vi "SL_0.vi"   [LabVIEW 2015, in "Lego_Swerve_2015.lvrbt"]
uses:
  Lego_Swerve_2015.lvrbt
  <vilib>/NXT/Block Support/NXT_OutputPort.ctl
  <vilib>/NXT/Block Support/NXT_MessageMailbox.ctl
  <vilib>/NXT/NXTIO Xnodes/NXTIONodeSubVIs/LEGOResetMotors.vi
  <vilib>/NXT/Dual Mode Library/Motors/Rotation.vi
  <vilib>/NXT/NXTIO Xnodes/NXTIONodeSubVIs/LEGOMotorStatus.vi
  <vilib>/NXT/Dual Mode Library/Display/drawNumber.vi
  <vilib>/NXT/Dual Mode Library/BT/BlueTooth_Read_string.vi
  <vilib>/NXT/NXTIO Xnodes/NXTIONodeSubVIs/NXTMoveMotors.vi
  <vilib>/NXT/Dual Mode Library/Display/drawText.vi
  <vilib>/NXT/Subs/LVHSConnector.ctl
  <vilib>/NXT/NXTIO Xnodes/AddressXNode/NXTIOAddress.xnode
  <vilib>/NXT/NXTIO Xnodes/NXTIOXNode/NXTIO.xnode
  <vilib>/NXT/LegoClasses/BrickReference/BrickReference.lvclass
types:
  T1 = typedef "NXT_OutputPort.ctl" = u8
  T2 = typedef "LVHSConnector.ctl" = refnum<class "BrickReference.lvclass">
  T3 = typedef "NXT_MessageMailbox.ctl" = u8
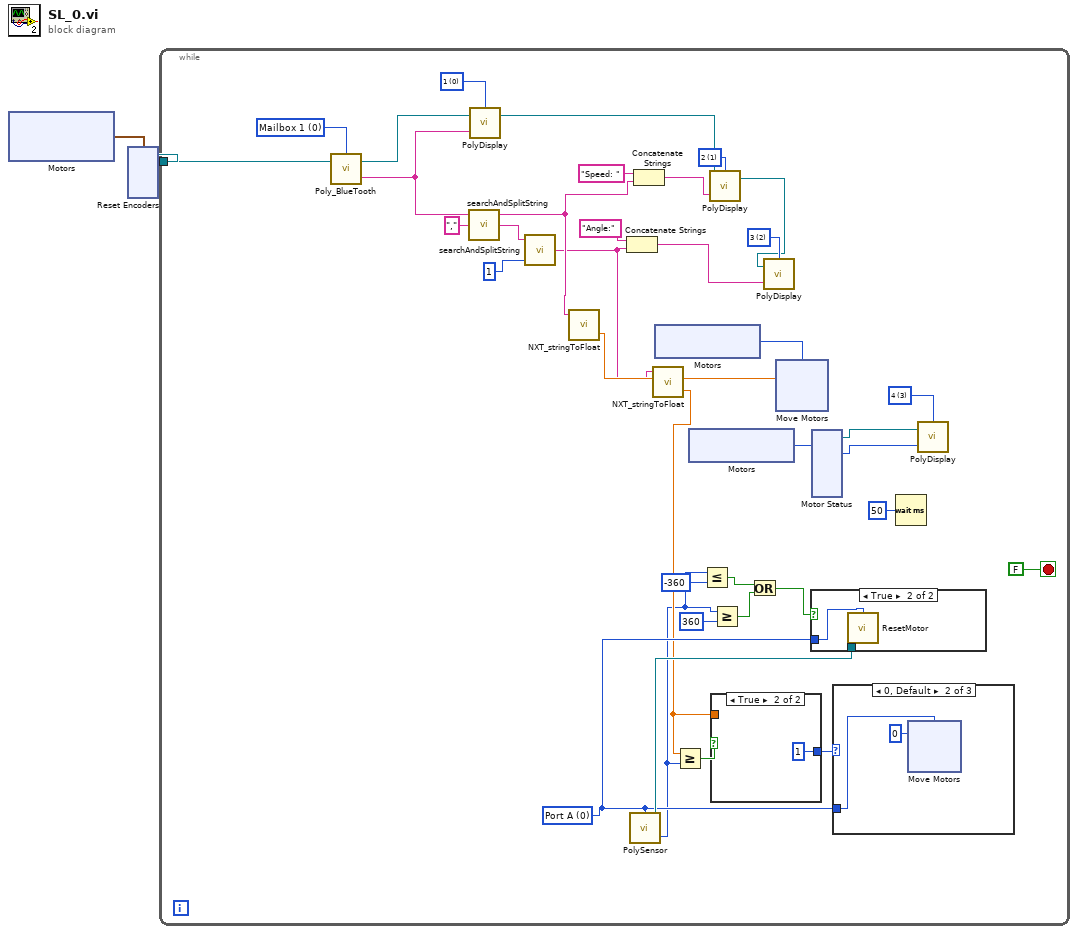
[diagram p0: block diagram]
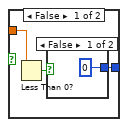
[diagram p2: hidden frame]
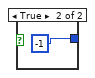
[diagram p3: hidden frame]
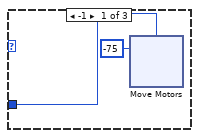
[diagram p5: hidden frame]
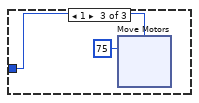
[diagram p6: hidden frame]
diagram:
  n1 = xnode "Motors"() -> ("Motor"=w1:cluster{"Port":T1, "Port":T1})
  n2 = xnode "Reset Encoders"("Motors"=w1) -> ("NXT/EV3"=w2:T2)  [unwired: 1 in]
  n3 = while {
    tunnel: w2 -> [w18]
    stop <- FALSE stop-if-true
    w11 = T1 0 items=["Port A", "Port B", "Port C", "Port D"] ("Port (Port A)")
    w16 = i16 3 items=["1", "2", "3", "4", "5", "6", "7", "8", "9", "10", "11", "12"] ("Line")
    w33 = i16 1 items=["1", "2", "3", "4", "5", "6", "7", "8", "9", "10", "11", "12"] ("Line")
    w34 = i16 2 items=["1", "2", "3", "4", "5", "6", "7", "8", "9", "10", "11", "12"] ("Line")
    w35 = i16 0 items=["1", "2", "3", "4", "5", "6", "7", "8", "9", "10", "11", "12"] ("Line")
    w37 = T3 0 items=["Mailbox 1", "Mailbox 2", "Mailbox 3", "Mailbox 4", "Mailbox 5", "Mailbox 6", "Mailbox 7", "Mailbox 8", "Mailbox 9", "Mailbox 10"] ("Mailbox")
    n4 = call-poly <vilib>:"Poly_BlueTooth.vi"("NXT/EV3"=w18, "Mailbox"=w37) -> ("Message"=w38:string, "NXT/EV3"=w22:T2)  [unwired: 1 in]
    n5 = call <vilib>:"searchAndSplitString.vi"("search string/char (-)"=",", "string"=w38) -> ("match + rest of string"=w26:string, "substring before match"=w25:string)  [unwired: 1 in, 1 out]
    n6 = call-poly <vilib>:"PolyDisplay.vi"("Text"=w38, "NXT/EV3"=w22, "Line"=w35) -> ("NXT/EV3"=w21:T2)  [unwired: 1 in]
    n7 = call <vilib>:"searchAndSplitString.vi"("offset (0)"=1, "string"=w26) -> ("match + rest of string"=w23:string)  [unwired: 1 in, 2 out]
    n8 = call <vilib>:"NXT_stringToFloat.vi"("string"=w25) -> ("number"=w24:sgl)  [unwired: 2 in, 1 out]
    n9 = Concatenate Strings("Angle:" ("string"), w23) -> (w30:string)
    n10 = call-poly <vilib>:"PolySensor.vi"("Port (Port A)"=w11) -> ("Angle of Rotation"=w4:i32, "NXT/EV3"=w13:T2)  [unwired: 2 in]
    n11 = Concatenate Strings("Speed: " ("string"), w25) -> (w32:string)
    n12 = call <vilib>:"NXT_stringToFloat.vi"("string"=w23) -> ("number"=w8:sgl)  [unwired: 2 in, 1 out]
    n13 = xnode "Motors"() -> ("Motor"=w28:T1)
    n14 = Greater Or Equal?(x=w8, y=w4) -> (x >= y?=w10:bool)
    n15 = xnode "Motors"() -> ("Motor"=w14:T1)
    n16 = Less Or Equal?(x=w4, y=-360) -> (x <= y?=w5:bool)
    n17 = call-poly <vilib>:"PolyDisplay.vi"("Text"=w32, "NXT/EV3"=w21, "Line"=w33) -> ("NXT/EV3"=w20:T2)  [unwired: 1 in]
    n18 = case shown="True" w10 {
      tunnel: [w42 1] -> w9
      tunnel: w8 -> [w40 _]
      frame False {
        n19 = Less Than 0?(x=w40) -> (x < 0?=w41:bool)
        n20 = case shown="False" w41 {
          tunnel: [0 -1] -> w42
          frame False {
          }
          frame True {
          }
        }
      }
      frame True {
      }
    }
    n21 = Greater Or Equal?(x=w4, y=360) -> (x >= y?=w7:bool)
    n22 = Or(x=w5, y=w7) -> (x .or. y?=w6:bool)
    n23 = call-poly <vilib>:"PolyDisplay.vi"("Text"=w30, "NXT/EV3"=w20, "Line"=w34) -> ()  [unwired: 1 in, 1 out]
    n24 = xnode "Move Motors"("Power/Speed 1"=w24, "Motors"=w28) -> ()  [unwired: 1 in, 1 out]
    n25 = case shown="True" w6 {
      tunnel: w13 -> [_ w47]
      tunnel: w11 -> [_ w46]
      frame False {
      }
      frame True {
        n26 = call <vilib>:"ResetMotor.vi"("NXT/EV3"=w47, "Port (All Ports)"=w46) -> ()  [unwired: 2 in, 1 out]
      }
    }
    n27 = xnode "Motor Status"("Motors"=w14) -> ("Position 1"=w17:i32, "NXT/EV3"=w15:T2)  [unwired: 1 in, 1 out]
    n28 = case shown="0, Default" w9 {
      tunnel: w11 -> [w48 w57 w66]
      frame -1 {
        n29 = xnode "Move Motors"("Power/Speed 1"=i8 -75, "Motors"=w48) -> ()  [unwired: 1 in, 1 out]
      }
      frame 0, Default {
        n30 = xnode "Move Motors"("Power/Speed 1"=i8 0, "Motors"=w57) -> ()  [unwired: 1 in, 1 out]
      }
      frame 1 {
        n31 = xnode "Move Motors"("Power/Speed 1"=i8 75, "Motors"=w66) -> ()  [unwired: 1 in, 1 out]
      }
    }
    n32 = Wait (ms)(milliseconds to wait=u32 50) -> ()  [unwired: 1 out]
    n33 = call-poly <vilib>:"PolyDisplay.vi"("number"=w17, "NXT/EV3"=w15, "Line"=w16) -> ()  [unwired: 1 in, 1 out]
  }
